vi "Check for Contact.vi"(8 "error in (no error)":errorcluster, 11 "Game Engine in":refnum<class "Game Engine.lvclass">) -> (0 "error out":errorcluster, 1 "Contact":bool, 3 "Game Engine out":refnum<class "Game Engine.lvclass">)   [LabVIEW 2017, in "Game Engine.lvlib" / "Game Engine.lvclass"]
uses:
  Game Engine.lvclass
  Game Engine.lvclass/Game Engine.ctl
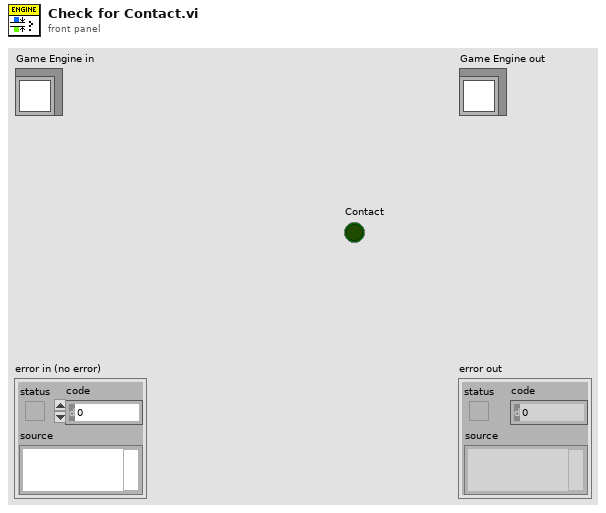
[diagram p1: front panel]
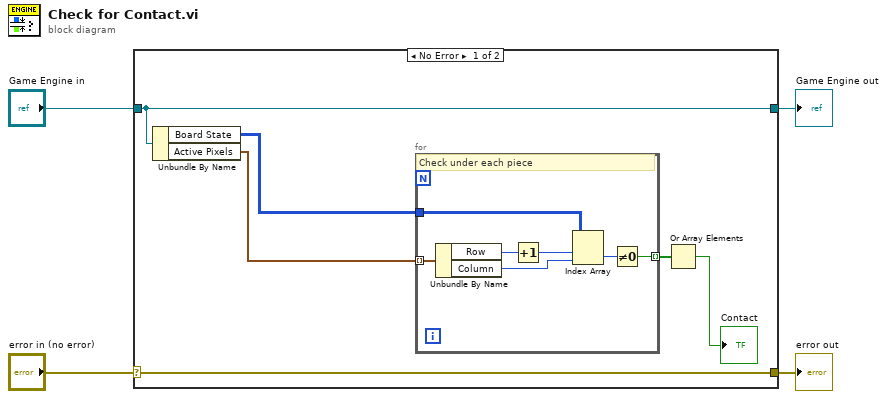
[diagram p0: block diagram]
diagram:
  n1 = case shown="No Error" "error in (no error)" {
    selector: "error in (no error)" -> [w10 w19]
    tunnel: [w10 w19] -> w3
    tunnel: [w8 w18] -> w1
    tunnel: "Game Engine in" -> [w8 w18]
    frame No Error {
      n2 = Unbundle By Name(w8) -> ("Board State"=w5:u32[][], "Active Pixels"=w9:cluster{"Column":u8, "Row":u8, "Color":u32}[])
      n3 = for {
        tunnel: w9 -> [w17] mode=indexing
        tunnel: w5 -> [w16]
        tunnel: [w11] -> w7 mode=indexing
        # "Check under each piece"
        n4 = Unbundle By Name(w17) -> ("Row"=w14:u8, "Column"=w15:u8)
        n5 = Increment(x=w14) -> (x+1=w13:u8)
        n6 = Index Array(array=w16, index (row)=w13, index (col)=w15) -> (element=w12:u32)
        n7 = Not Equal To 0?(x=w12) -> (x != 0?=w11:bool)
      }
      n8 = Or Array Elements(Boolean array=w7) -> (logical OR=→"Contact":bool)
    }
    frame Error {
    }
  }
  "error out" <- w3
  "Game Engine out" <- w1
